vi "Actor Core.vi"(8 "error in":errorcluster, 11 "SwitchMatrix in":refnum<class "SwitchMatrix.lvclass">) -> (0 "error out":errorcluster, 3 "Actor out":refnum<class "Actor.lvclass">)   [LabVIEW 2019, in "SwitchMatrix.lvlib" / "SwitchMatrix.lvclass"]
doc: "The instrument actor core is only here to distribute panel resolution settings to children classes."
uses:
  Library/SwitchMatrix.lvclass
  builds/Engine/Actor Framework.lvlibp/1abvi3w/vi.lib/ActorFramework/Actor/Actor.lvclass
  Library/SwitchMatrix.lvclass/SwitchMatrix.ctl
  SwitchMatrix Messages/Toggle Relay Msg/Toggle Relay Msg.lvclass/Toggle Relay Msg.ctl
  Private/Accessors/Write Display_Ref.vi
  builds/Engine/Actor Framework.lvlibp/1abvi3w/vi.lib/ActorFramework/Message Enqueuer/Enqueue.vi
  SwitchMatrix Messages/Toggle Relay Msg/Toggle Relay Msg.lvclass
  SwitchMatrix Messages/Open All Relays Msg/Open All Relays Msg.lvclass
  builds/Instruments/Instruments.lvlibp/Library/Instruments.lvclass
  C:/Users/Public/Documents/Development/builds/Instruments/Instruments.lvlibp/Library/Instruments.lvclass
panel:
  in  "Clear All":bool
  in  "Active Device":u16(ring)
  in  "Topology":T1(tab)
  in  "Unroute 1 0":bool
  in  "Route 1 0":bool
  in  "Single_ind_0":i32(listbox)
  in  "Single_ctl_0":i32(listbox)
  in  "Unroute 2 1":bool
  in  "Route 2 1":bool
  in  "Unroute 2 0":bool
  in  "Route 2 0":bool
  in  "Dual_ind_1":i32(listbox)
  in  "Dual_ind_0":i32(listbox)
  in  "Dual_ctl_1":i32(listbox)
  in  "Dual_ctl_0":i32(listbox)
  in  "Unroute 4 3":bool
  in  "Route 4 3":bool
  in  "Quad_ind_3":i32(listbox)
  in  "Quad_ctl_3":i32(listbox)
  in  "Unroute 4 2":bool
  in  "Route 4 2":bool
  in  "Quad_ind_2":i32(listbox)
  in  "Quad_ctl_2":i32(listbox)
  in  "Unroute 4 1":bool
  in  "Route 4 1":bool
  in  "Quad_ind_1":i32(listbox)
  in  "Quad_ctl_1":i32(listbox)
  in  "Unroute 4 0":bool
  in  "Route 4 0":bool
  in  "Quad_ind_0":i32(listbox)
  in  "Quad_ctl_0":i32(listbox)
  in  "Unroute 8 7":bool
  in  "Route 8 7":bool
  in  "Octal_ind_h":i32(listbox)
  in  "Octal_ctl_i":i32(listbox)
  in  "Unroute 8 6":bool
  in  "Route 8 6":bool
  in  "Octal_ind_g":i32(listbox)
  in  "Octal_ctl_g":i32(listbox)
  in  "Unroute 8 5":bool
  in  "Route 8 5":bool
  in  "Octal_ind_f":i32(listbox)
  in  "Octal_ctl_f":i32(listbox)
  in  "Unroute 8 4":bool
  in  "Route 8 4":bool
  in  "Octal_ind_e":i32(listbox)
  in  "Octal_ctl_e":i32(listbox)
  in  "Unroute 8 3":bool
  in  "Route 8 3":bool
  in  "Octal_ind_d":i32(listbox)
  in  "Octal_ctl_d":i32(listbox)
  in  "Unroute 8 2":bool
  in  "Route 8 2":bool
  in  "Octal_ind_c":i32(listbox)
  in  "Octal_ctl_c":i32(listbox)
  in  "Unroute 8 1":bool
  in  "Route 8 1":bool
  in  "Octal_ind_b":i32(listbox)
  in  "Octal_ctl_b":i32(listbox)
  in  "Unroute 8 0":bool
  in  "Route 8 0":bool
  in  "Octal_ind_a":i32(listbox)
  in  "Octal_ctl_a":i32(listbox)
  in  "Unroute 16 15":bool
  in  "Route 16 15":bool
  in  "sxtn_ind_p":i32(listbox)
  in  "sxtn_ctl_p":i32(listbox)
  in  "Unroute 16 14":bool
  in  "Route 16 14":bool
  in  "sxtn_ind_o":i32(listbox)
  in  "sxtn_ctl_o":i32(listbox)
  in  "Unroute 16 13":bool
  in  "Route 16 13":bool
  in  "sxtn_ind_n":i32(listbox)
  in  "sxtn_ctl_n":i32(listbox)
  in  "Unroute 16 12":bool
  in  "Route 16 12":bool
  in  "sxtn_ind_m":i32(listbox)
  in  "sxtn_ctl_m":i32(listbox)
  in  "Unroute 16 11":bool
  in  "Route 16 11":bool
  in  "sxtn_ind_l":i32(listbox)
  in  "sxtn_ctl_l":i32(listbox)
  in  "Unroute 16 10":bool
  in  "Route 16 10":bool
  in  "sxtn_ind_k":i32(listbox)
  in  "sxtn_ctl_k":i32(listbox)
  in  "Unroute 16 9":bool
  in  "Route 16 9":bool
  in  "sxtn_ind_j":i32(listbox)
  in  "sxtn_ctl_j":i32(listbox)
  in  "Unroute 16 8":bool
  in  "Route 16 8":bool
  in  "sxtn_ind_i":i32(listbox)
  in  "sxtn_ctl_i":i32(listbox)
  in  "Unroute 16 7":bool
  in  "Route 16 7":bool
  in  "sxtn_ind_h":i32(listbox)
  in  "sxtn_ctl_h":i32(listbox)
  in  "Unroute 16 6":bool
  in  "Route 16 6":bool
  in  "sxtn_ind_g":i32(listbox)
  in  "sxtn_ctl_g":i32(listbox)
  in  "Unroute 16 5":bool
  in  "Route 16 5":bool
  in  "sxtn_ind_f":i32(listbox)
  in  "sxtn_ctl_e":i32(listbox)
  in  "Unroute 16 4":bool
  in  "Route 16 4":bool
  in  "sxtn_ind_e":i32(listbox)
  in  "sxtn_ctl_f":i32(listbox)
  in  "Unroute 16 3":bool
  in  "Route 16 3":bool
  in  "sxtn_ind_d":i32(listbox)
  in  "sxtn_ctl_d":i32(listbox)
  in  "Unroute 16 2":bool
  in  "Route 16 2":bool
  in  "sxtn_ind_c":i32(listbox)
  in  "sxtn_ctl_c":i32(listbox)
  in  "Unroute 16 1":bool
  in  "Route 16 1":bool
  in  "sxtn_ind_b":i32(listbox)
  in  "sxtn_ctl_b":i32(listbox)
  in  "Unroute 16 0":bool
  in  "Route 16 0":bool
  in  "sxtn_ind_a":i32(listbox)
  in  "sxtn_ctl_a":i32(listbox)
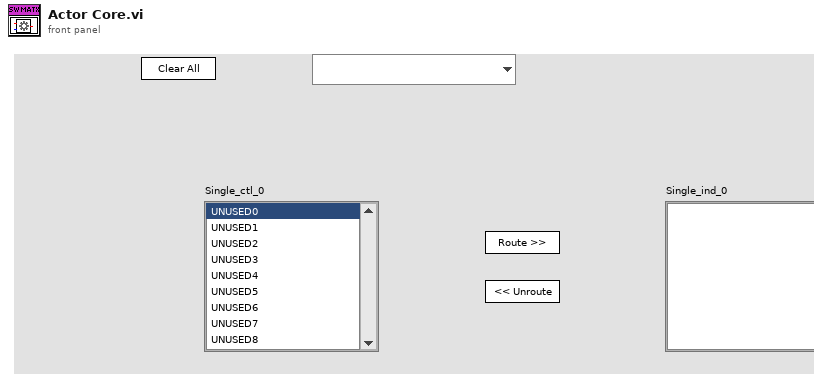
[diagram p1: front panel]
types:
  T1 = enum32{"Single", "Dual", "Quad", "Octal", "Sixteen"}
  T2 = cluster{"Pnl Actor":refnum<event-registration>, "Event Registration Refnum":refnum<event-registration>}
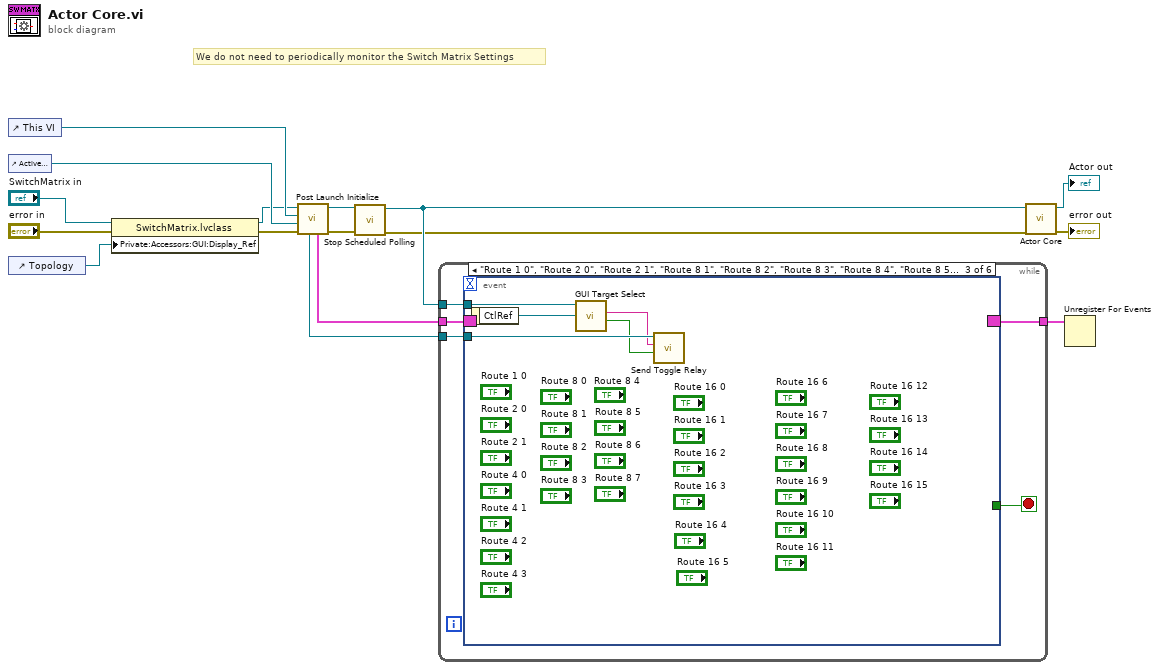
[diagram p0: block diagram]
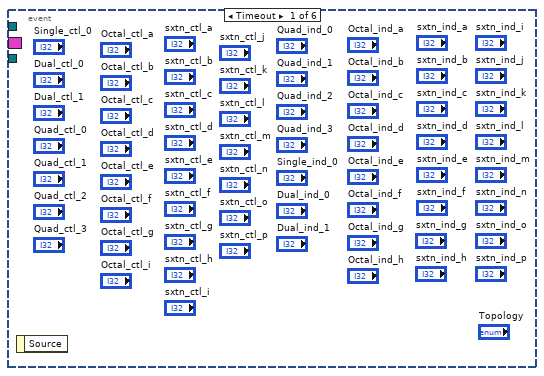
[diagram p2: hidden frame]
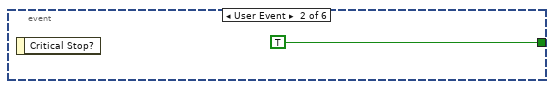
[diagram p3: hidden frame]
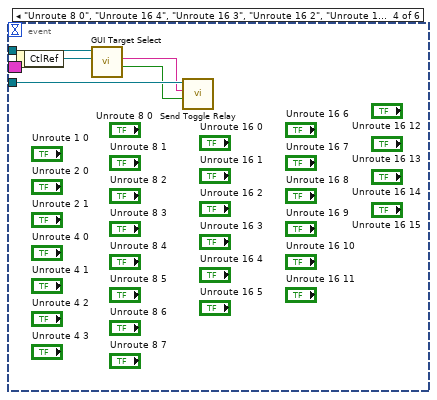
[diagram p4: hidden frame]
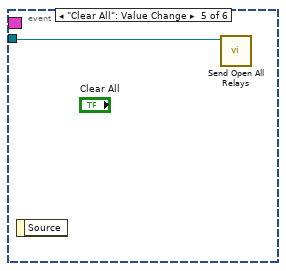
[diagram p5: hidden frame]
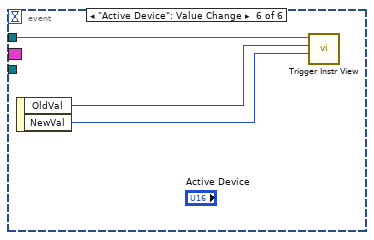
[diagram p6: hidden frame]
diagram:
  # "We do not need to periodically monitor the Switch Matrix Settings"
  n1 = control-ref of="This VI"() -> (w12:refnum<vi>)
  n2 = control-ref of="Active Device"() -> (w11:refnum<vi>)
  n3 = control-ref of="Topology"() -> (w6:refnum<vi>)
  n4 = property class="SwitchMatrix.lvclass"(reference="SwitchMatrix in", error in="error in", "Private:Accessors:GUI:Display_Ref"=w6) -> (reference out=w7:refnum<class "SwitchMatrix.lvclass">, error out=w8:errorcluster)
  n5 = call "Post Launch Initialize.vi"("error in"=w8, "Active Device"=w11, "GUI Reference"=w12, "Instruments in"=w7) -> ("error out"=w4:errorcluster, "Instruments out"=w3:refnum<class "SwitchMatrix.lvclass">, "Registered Events"=w14:T2, "Self Enqueuer"=w13:refnum<class "Message Enqueuer.lvclass">)  [unwired: 4 in]
  n6 = call "Stop Scheduled Polling.vi"("error in"=w4, "Instruments in"=w3) -> ("error out"=w1:errorcluster, "Instruments out"=w2:refnum<class "SwitchMatrix.lvclass">)  [unwired: 8 in]
  n7 = while {
    tunnel: w14 -> [w21]
    tunnel: w13 -> [w18]
    tunnel: w2 -> [w17]
    tunnel: [w20] -> w10
    stop <- w19 stop-if-true
    n8 = event shown="[2] \"Route 1 0\", \"Route 2 0\", \"Route 2 1\", \"Route 8 1\", \"Route 8 2\", \"Route 8 3\", \"Route 8 4\", \"Route 8 5\", \"Route 8 6\", \"Route 8 7\", \"Route 4 0\", \"Route 4 1\", \"Route 4 2\", \"Route 4 3\", \"Route 16 0\", \"Route 16 1\", \"Route 16 2\", \"Route 16 3\", \"Route 16 4\", \"Route 16 5\", \"Route 16 6\", \"Route 16 7\", \"Route 16 8\", \"Route 16 9\", \"Route 16 10\", \"Route 16 11\", \"Route 16 12\", \"Route 16 13\", \"Route 16 14\", \"Route 16 15\", \"Route 8 0\": Value Change" {
      selector: w21 -> [_ _ _ _ _ _]
      dyn-events: [_ _ _ _ _ _] -> w20
      timeout: _ -> [_ _ _ _ _ _]
      tunnel: [_ TRUE _ _ _ _] -> w19
      tunnel: w18 -> [_ _ w27 w30 w33 _]
      tunnel: w17 -> [_ _ w26 w31 _ w36]
      event Timeout {
        n9 = event-data() -> ()  [unwired: 1 in, 1 out]
      }
      event User Event {
        n10 = event-data() -> ()  [unwired: 1 in, 1 out]
      }
      event "Route 1 0", "Route 2 0", "Route 2 1", "Route 8 1", "Route 8 2", "Route 8 3", "Route 8 4", "Route 8 5", "Route 8 6", "Route 8 7", "Route 4 0", "Route 4 1", "Route 4 2", "Route 4 3", "Route 16 0", "Route 16 1", "Route 16 2", "Route 16 3", "Route 16 4", "Route 16 5", "Route 16 6", "Route 16 7", "Route 16 8", "Route 16 9", "Route 16 10", "Route 16 11", "Route 16 12", "Route 16 13", "Route 16 14", "Route 16 15", "Route 8 0": Value Change {
        n11 = event-data() -> ("CtlRef"=w25:refnum<vi>)  [unwired: 1 in]
        n12 = call "GUI Target Select.vi"("Control_Reference"=w25, "SwitchMatrix in"=w26) -> ("Value"=w23:bool, "Target"=w24:string)  [unwired: 6 in, 2 out]
        n13 = call "Send Toggle Relay.vi"("Relay State"=w23, "Relay Name"=w24, "Message Enqueuer"=w27) -> ()  [unwired: 7 in, 2 out]
      }
      event "Unroute 8 0", "Unroute 16 4", "Unroute 16 3", "Unroute 16 2", "Unroute 16 1", "Unroute 16 0", "Unroute 16 5", "Unroute 16 6", "Unroute 16 7", "Unroute 16 8", "Unroute 16 9", "Unroute 16 10", "Unroute 16 11", "Unroute 16 12", "Unroute 16 13", "Unroute 16 14", "Unroute 16 15", "Unroute 4 1", "Unroute 4 0", "Unroute 4 2", "Unroute 4 3", "Unroute 1 0", "Unroute 2 0", "Unroute 2 1", "Unroute 8 1", "Unroute 8 2", "Unroute 8 3", "Unroute 8 4", "Unroute 8 5", "Unroute 8 6", "Unroute 8 7": Value Change {
        n14 = event-data() -> ("CtlRef"=w32:refnum<vi>)  [unwired: 1 in]
        n15 = call "GUI Target Select.vi"("Control_Reference"=w32, "SwitchMatrix in"=w31) -> ("Value"=w28:bool, "Target"=w29:string)  [unwired: 6 in, 2 out]
        n16 = call "Send Toggle Relay.vi"("Relay State"=w28, "Relay Name"=w29, "Message Enqueuer"=w30) -> ()  [unwired: 7 in, 2 out]
      }
      event "Clear All": Value Change {
        n17 = event-data() -> ()  [unwired: 1 in, 1 out]
        n18 = call "Send Open All Relays.vi"("Message Enqueuer"=w33) -> ()  [unwired: 9 in, 2 out]
      }
      event "Active Device": Value Change {
        n19 = event-data() -> ("OldVal"=w35:u16, "NewVal"=w34:u16)  [unwired: 1 in]
        n20 = call "Trigger Instr View.vi"("New Value"=w34, "Old Value"=w35, "Instruments in"=w36) -> ()  [unwired: 7 in, 2 out]
      }
    }
  }
  n21 = call-parent "Actor Core.vi"("error in"=w1, "Instruments in"=w2) -> ("error out"=→"error out":errorcluster, "Actor out"=→"Actor out":refnum<class "Actor.lvclass">)  [unwired: 8 in]
  n22 = Unregister For Events(event registration refnum=w10) -> ()  [unwired: 1 in, 1 out]
